vi "CommandRecieve.vi"(8 "error in (no error)":errorcluster, 9 "Mission Notifiers":T1, 10 "NotifierReff":T2, 11 "NetworkStreamReader in":refnum<class "NetworkStreamReader.lvclass">) -> (0 "error out":errorcluster, 2 "NetworkStreamReader out":refnum<class "NetworkStreamReader.lvclass">)   [LabVIEW 2013]
doc: "Recieves the Mission data from the OCU and stroes it in the Reciecved Missions Queue\n\nElizabeth Mahon and Victoria\n01/14"
uses:
  RIO-OCU_Comm/NetworkStreams/Reader/NetworkStreamReader.lvclass
  Data/TypeDefs/Notifiers.ctl
  Data/TypeDefs/UTM Location.ctl
  Data/TypeDefs/Sail Set Suggestions.ctl
  Data/TypeDefs/Rudder Set Suggestions.ctl
  Data/TypeDefs/OverrideInformation.ctl
  Data/TypeDefs/OverrideMode.ctl
  Data/TypeDefs/MotorSetup.ctl
  Data/TypeDefs/DynamixelSetupInfo.ctl
  Data/TypeDefs/AirmarStatus.ctl
  Data/TypeDefs/HardwareOnline.ctl
  Data/TypeDefs/DynamixelCycleTracker.ctl
  Data/TypeDefs/RC Input Values.ctl
  Classes/Waypoint/Waypoint.lvclass
  Data/TypeDefs/MissionNotifiers.ctl
  Classes/Missions/GenericMission/GenericMission.lvclass
  Classes/Obstacle/Obstacle.lvclass
  RIO-OCU_Comm/ToRIO.ctl
  OCU/CommandMessages.ctl
  Data/TypeDefs/Constants for OCU Tuning.ctl
panel:
  out "Connected?":bool
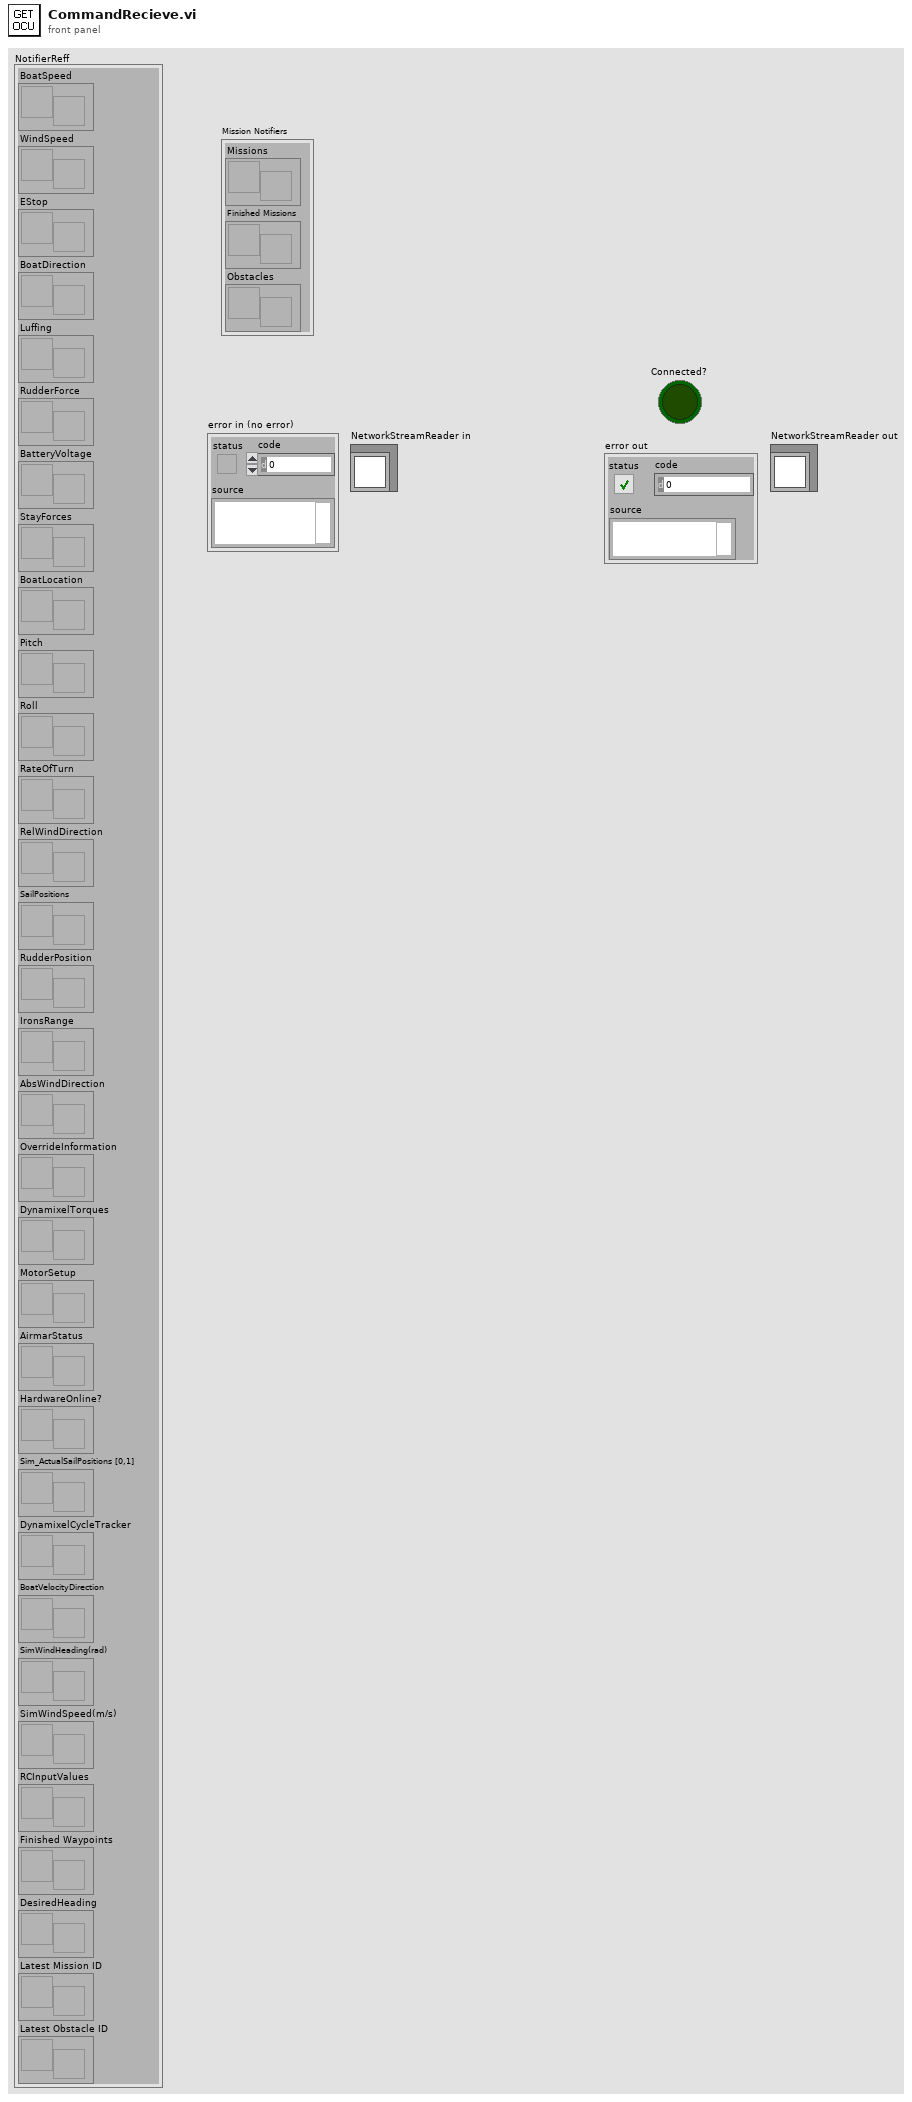
[diagram p1: front panel]
types:
  T1 = typedef "MissionNotifiers.ctl" = cluster{"Missions":refnum<notifier>, "Finished Missions":refnum<notifier>, "Obstacles":refnum<notifier>}
  T2 = typedef "Notifiers.ctl" = cluster{"BoatSpeed":refnum<notifier>, "WindSpeed":refnum<notifier>, "EStop":refnum<notifier>, "BoatDirection":refnum<notifier>, "Luffing":refnum<notifier>, "RudderForce":refnum<notifier>, "BatteryVoltage":refnum<notifier>, "StayForces":refnum<notifier>, "BoatLocation":refnum<notifier>, "Pitch":refnum<notifier>, "Roll":refnum<notifier>, "RateOfTurn":refnum<notifier>, "RelWindDirection":refnum<notifier>, "SailPositions":refnum<notifier>, "RudderPosition":refnum<notifier>, "IronsRange":refnum<notifier>, "AbsWindDirection":refnum<notifier>, "OverrideInformation":refnum<notifier>, "DynamixelTorques":refnum<notifier>, "MotorSetup":refnum<notifier>, "AirmarStatus":refnum<notifier>, "HardwareOnline?":refnum<notifier>, "Sim_ActualSailPositions [0,1]":refnum<notifier>, "DynamixelCycleTracker":refnum<notifier>, "BoatVelocityDirection":refnum<notifier>, "SimWindHeading(rad)":refnum<notifier>, "SimWindSpeed(m/s)":refnum<notifier>, "RCInputValues":refnum<notifier>, "Finished Waypoints":refnum<notifier>, "DesiredHeading":refnum<notifier>, "Latest Mission ID":refnum<notifier>, "Latest Obstacle ID":refnum<notifier>}
  T3 = typedef "ToRIO.ctl" = cluster{"Commands":T4, "Variant":variant}
  T4 = typedef "CommandMessages.ctl" = enum16{"Pass", "OverrideMode", "Add mission", "Delete mission", "Add obstacle", "Delete obstacle", "Change constants", "Check mission ID", "Check obstacle ID"}
  T5 = typedef "OverrideInformation.ctl" = cluster{"OverrideMode":T6, "SailSetting":T7, "Rudder Setpoint":T8, "Sim_Wind_Speed":dbl, "Sim_Wind_Heading":dbl}
  T6 = typedef "OverrideMode.ctl" = enum16{"None", "Rudder", "Sails", "Both"}
  T7 = typedef "Sail Set Suggestions.ctl" = cluster{"MainSailSuggestion":dbl, "JibSailSuggestion":dbl}
  T8 = typedef "Rudder Set Suggestions.ctl" = dbl
  T9 = typedef "Constants for OCU Tuning.ctl" = cluster{"Motor Setting Constant":T10, "Irons Range (deg)":dbl}
  T10 = typedef "MotorSetup.ctl" = cluster{"Main Dynamixel Set Data":T11, "Rudder Dynamixel Set Data":T11, "Jib Dynamixel Set Data":T11}
  T11 = typedef "DynamixelSetupInfo.ctl" = cluster{"Lower Winch Bound (deg)":dbl, "Upper Winch Bound (deg)":dbl}
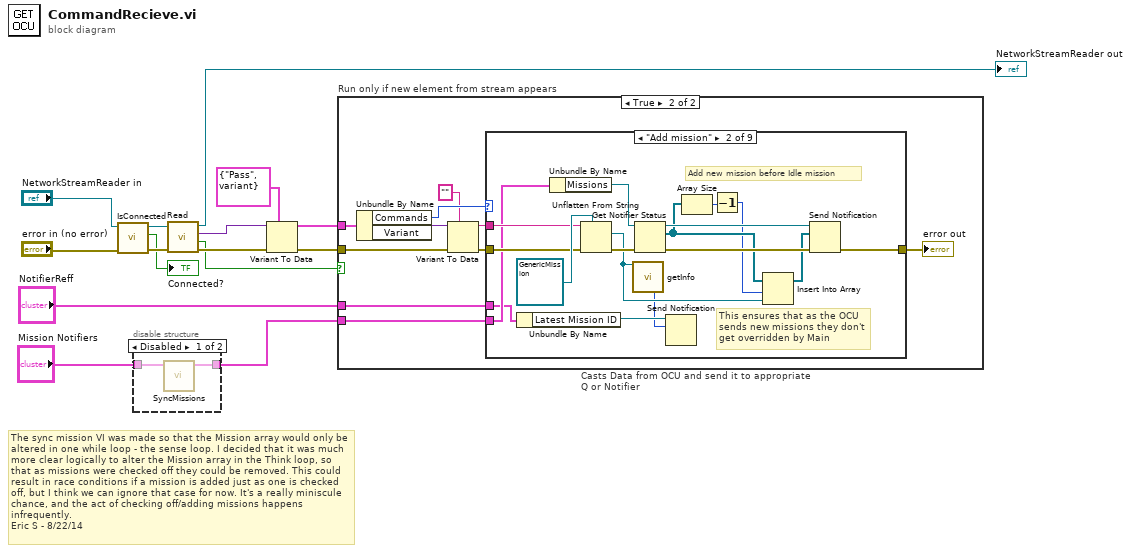
[diagram p0: block diagram]
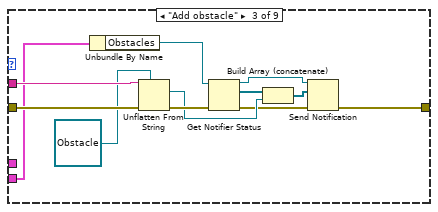
[diagram p5: hidden frame]
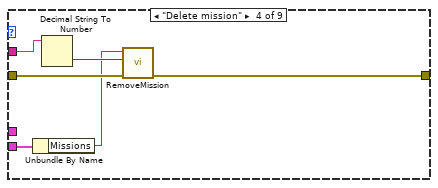
[diagram p6: hidden frame]
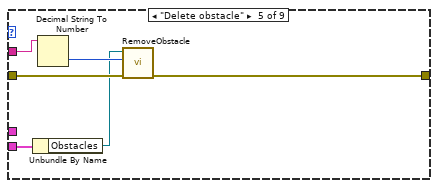
[diagram p7: hidden frame]
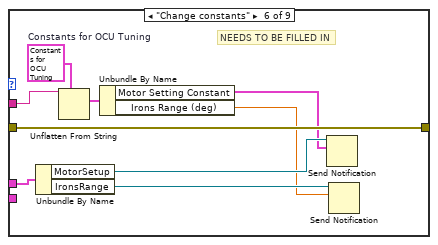
[diagram p8: hidden frame]
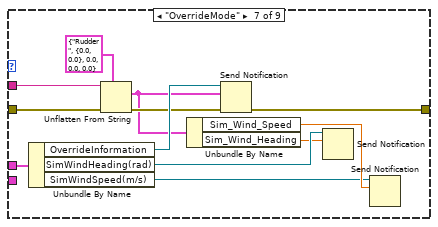
[diagram p9: hidden frame]
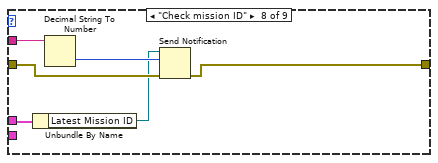
[diagram p10: hidden frame]
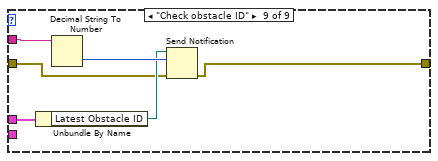
[diagram p11: hidden frame]
diagram:
  # "The sync mission VI was made so that the Mission array would only be altered in one while loop - the sense loop. I decided that it was much more clear logically to alter the Mission array in the Think loop, so that as missions were checked off they could be removed. This could result in race conditions if a mission is added just as one is checked off, but I think we can ignore that case for now. It's a really miniscule chance, and the act of checking off/adding missions happens infrequently.\nEric S - 8/22/14"
  n1 = call "IsConnected.vi"("error in (no error)"="error in (no error)", "NetworkStreamReader in"="NetworkStreamReader in") -> ("error out"=w8:errorcluster, "Connected?"=→"Connected?":bool, "NetworkStreamReader out"=w9:refnum<class "NetworkStreamReader.lvclass">)  [unwired: 7 in]
  n2 = disable-structure shown="Disabled" {
    disable-tunnel: "Mission Notifiers" -> [w17 w18]
    disable-tunnel: [w16 w18] -> w1
    frame Disabled {
      n3 = call "SyncMissions.vi"("Mission Notifiers"=w17) -> ("Mission Notifiers OUT"=w16:T1)  [unwired: 10 in]
    }
    frame Enabled {
    }
  }
  n4 = call "Read.vi"("error in (no error)"=w8, "NetworkStreamReader in"=w9) -> ("error out"=w13:errorcluster, "New element?"=w3:bool, "element"=w4:variant, "NetworkStreamReader out"=→"NetworkStreamReader out":refnum<class "NetworkStreamReader.lvclass">)  [unwired: 5 in, 1 out]
  n5 = Variant To Data(error in=w13, type=T3 {"Commands"=enum."Pass", "Variant"=variant} ("To RIO"), Variant=w4) -> (data=w11:T3, error out=w12:errorcluster)
  n6 = case "Run only if new element from stream appears" shown="True" w3 {
    tunnel: w12 -> [_ w21]
    tunnel: w11 -> [_ w27]
    tunnel: "NotifierReff" -> [_ w25]
    tunnel: w1 -> [_ w19]
    frame False {
    }
    frame True {
      n7 = Unbundle By Name(w27) -> ("Commands"=w26:T4, "Variant"=w23:variant)
      n8 = Variant To Data(error in=w21, type="", Variant=w23) -> (data=w22:string, error out=w20:errorcluster)
      n9 = case "Casts Data from OCU and send it to appropriate Q or Notifier" shown="\"Add mission\"" w26 {
        tunnel: w20 -> [w29 w41 w57 w62 w69 w79 w90 w95 w101]
        tunnel: [w29 w40 w49 w61 w67 w79 w87 w92 w100] -> w28
        tunnel: w25 -> [_ w32 _ _ _ w75 w89 w96 w98]
        tunnel: w22 -> [_ w42 w58 w64 w70 w78 w85 w97 w99]
        tunnel: w19 -> [_ w39 w48 w60 w66 _ _ _ _]
        frame "Pass", Default {
        }
        frame "Add mission" {
          # "This ensures that as the OCU sends new missions they don't get overridden by Main"
          # "Add new mission before Idle mission"
          n10 = Unbundle By Name(w32) -> ("Latest Mission ID"=w31:refnum<notifier>)
          n11 = Unbundle By Name(w39) -> ("Missions"=w38:refnum<notifier>)
          n12 = Unflatten From String(type=refnum<class "GenericMission.lvclass"> refnum ("GenericMission in"), binary string=w42, error in (no error)=w41) -> (value=w33:refnum<class "GenericMission.lvclass">, error out=w46:errorcluster)  [unwired: 2 in, 1 out]
          n13 = call-dynamic "getInfo.vi"("GenericMission in"=w33) -> ("ID#"=w30:i16)  [unwired: 6 in, 8 out]
          n14 = Get Notifier Status(notifier=w38, error in (no error)=w46) -> (notifier out=w44:refnum<notifier>, current notification=w36:refnum<class "GenericMission.lvclass">[], error out=w45:errorcluster)  [unwired: 2 out]
          n15 = Send Notification(notification=w30, notifier=w31) -> ()  [unwired: 1 in, 2 out]
          n16 = Array Size(array=w36) -> (size(s)=w37:i32)
          n17 = Decrement(x=w37) -> (x-1=w35:i32)
          n18 = Insert Into Array(array=w36, index=w35, new element=w33) -> (w34:refnum<class "GenericMission.lvclass">[])
          n19 = Send Notification(notification=w34, notifier=w44, error in (no error)=w45) -> (error out=w40:errorcluster)  [unwired: 1 out]
        }
        frame "Add obstacle" {
          n20 = Unbundle By Name(w48) -> ("Obstacles"=w47:refnum<notifier>)
          n21 = Unflatten From String(type=refnum<class "Obstacle.lvclass"> refnum ("Obstacle.lvclass"), binary string=w58, error in (no error)=w57) -> (value=w53:refnum<class "Obstacle.lvclass">, error out=w55:errorcluster)  [unwired: 2 in, 1 out]
          n22 = Get Notifier Status(notifier=w47, error in (no error)=w55) -> (notifier out=w51:refnum<notifier>, current notification=w54:refnum<class "Obstacle.lvclass">[], error out=w52:errorcluster)  [unwired: 2 out]
          n23 = Build Array (concatenate)(w54, w53) -> (w50:refnum<class "Obstacle.lvclass">[])
          n24 = Send Notification(notification=w50, notifier=w51, error in (no error)=w52) -> (error out=w49:errorcluster)  [unwired: 1 out]
        }
        frame "Delete mission" {
          n25 = Unbundle By Name(w60) -> ("Missions"=w59:refnum<notifier>)
          n26 = Decimal String To Number(string=w64) -> (number=w63:i32)  [unwired: 2 in, 1 out]
          n27 = call "RemoveMission.vi"("error in (no error)"=w62, "ID to delete"=w63, "Mission Notifier"=w59) -> ("error out"=w61:errorcluster)  [unwired: 8 in]
        }
        frame "Delete obstacle" {
          n28 = Unbundle By Name(w66) -> ("Obstacles"=w65:refnum<notifier>)
          n29 = Decimal String To Number(string=w70) -> (number=w68:i32)  [unwired: 2 in, 1 out]
          n30 = call "RemoveObstacle.vi"("error in (no error)"=w69, "ID to delete"=w68, "Obstacle Notifier"=w65) -> ("error out"=w67:errorcluster)  [unwired: 8 in]
        }
        frame "Change constants" {
          w77 = T9 {"Motor Setting Constant"={"Main Dynamixel Set Data"={"Lower Winch Bound (deg)"=0.0, "Upper Winch Bound (deg)"=0.0}, "Rudder Dynamixel Set Data"={"Lower Winch Bound (deg)"=0.0, "Upper Winch Bound (deg)"=0.0}, "Jib Dynamixel Set Data"={"Lower Winch Bound (deg)"=0.0, "Upper Winch Bound (deg)"=0.0}}, "Irons Range (deg)"=0.0}  # Constants for OCU Tuning
          # "NEEDS TO BE FILLED IN"
          n31 = Unbundle By Name(w75) -> ("MotorSetup"=w74:refnum<notifier>, "IronsRange"=w72:refnum<notifier>)
          n32 = Unflatten From String(type=w77, binary string=w78) -> (value=w76:T9)  [unwired: 3 in, 2 out]
          n33 = Unbundle By Name(w76) -> ("Motor Setting Constant"=w73:T10, "Irons Range (deg)"=w71:dbl)
          n34 = Send Notification(notification=w73, notifier=w74) -> ()  [unwired: 1 in, 2 out]
          n35 = Send Notification(notification=w71, notifier=w72) -> ()  [unwired: 1 in, 2 out]
        }
        frame "OverrideMode" {
          n36 = Unbundle By Name(w89) -> ("OverrideInformation"=w88:refnum<notifier>, "SimWindHeading(rad)"=w84:refnum<notifier>, "SimWindSpeed(m/s)"=w81:refnum<notifier>)
          n37 = Unflatten From String(type=T5 {"OverrideMode"=enum."Rudder", "SailSetting"={"MainSailSuggestion"=0.0, "JibSailSuggestion"=0.0}, "Rudder Setpoint"=0.0, "Sim_Wind_Speed"=0.0, "Sim_Wind_Heading"=0.0}, binary string=w85, error in (no error)=w90) -> (value=w80:T5, error out=w86:errorcluster)  [unwired: 2 in, 1 out]
          n38 = Unbundle By Name(w80) -> ("Sim_Wind_Speed"=w82:dbl, "Sim_Wind_Heading"=w83:dbl)
          n39 = Send Notification(notification=w80, notifier=w88, error in (no error)=w86) -> (error out=w87:errorcluster)  [unwired: 1 out]
          n40 = Send Notification(notification=w83, notifier=w84) -> ()  [unwired: 1 in, 2 out]
          n41 = Send Notification(notification=w82, notifier=w81) -> ()  [unwired: 1 in, 2 out]
        }
        frame "Check mission ID" {
          n42 = Unbundle By Name(w96) -> ("Latest Mission ID"=w93:refnum<notifier>)
          n43 = Decimal String To Number(string=w97) -> (number=w94:i32)  [unwired: 2 in, 1 out]
          n44 = Send Notification(notification=w94, notifier=w93, error in (no error)=w95) -> (error out=w92:errorcluster)  [unwired: 1 out]
        }
        frame "Check obstacle ID" {
          n45 = Unbundle By Name(w98) -> ("Latest Obstacle ID"=w102:refnum<notifier>)
          n46 = Decimal String To Number(string=w99) -> (number=w103:i32)  [unwired: 2 in, 1 out]
          n47 = Send Notification(notification=w103, notifier=w102, error in (no error)=w101) -> (error out=w100:errorcluster)  [unwired: 1 out]
        }
      }
      "error out" <- w28
    }
  }
